vi "SPARC4_GEI.vi"() -> ()   [LabVIEW 2018]
uses:
  S4GEI/SPARC4_GEI.lvclass
  S4GEI/SPARC4_GEI.lvclass/SPARC4_GEI.ctl
  FWCS_ACS_Iterator/FWCS_ACS_Iterator.lvclass/FWCS_ACS_Iterator.ctl
  Interface/Interface.lvclass/Interface.ctl
  Channel GUI/Channel.lvclass/Channel.ctl
  State Machine/State Machine.lvclass/State Machine.ctl
  Filter_Wheel/Filter_Wheel.lvclass/Filter_Wheel.ctl
  Channel GUI/Channel.lvclass
  FWCS_ACS_Iterator/FWCS_ACS_Iterator.lvclass
  State Machine/State Machine.lvclass
  Filter_Wheel/Filter_Wheel.lvclass
  RxTx/RxTx.lvclass
  Interface/Interface.lvclass
panel:
  in  "Tab Control 2":T1(tab)
  out "Frames done":u16(slide)=1 max=2 scale=0.0..1.0
  in  "Channel ID":u16=1 min=1
  in  "FOCUS":bool caption="TEST"
  in  "TEST":bool
  in  "ZERO":bool caption="BIAS"
  in  "FLAT":bool
  in  "OBJECT":bool caption="SCIENCE"
  in  "DARK":bool caption="TEST"
  in  "Suffix:":string
  in  "Comment:":string="Go SPARC4!"
  in  "Filter":u16(ring)=1 items=["U"=1, "B"=2, "V"=3, "R"=4, "I"=5, "Clear"=6]
  out "Cubes done":u16(slide)=1 max=2 scale=0.0..1.0
  out "Exposing":bool
  in  "Dummy":bool
  out "Camera On/Off":bool
  in  "Abort Acquisition":bool
  in  "Stop Acquisition":bool
  in  "#Cubes":u32=1 min=1
  in  "#Frames":u16=1 min=1 max=1000
  in  "Send Message":bool
  out "Response:":string
  in  "Command:":string
  out "Last image":string
  out "CCD Status":string
  out "Frame exp time (s)":dbl
  out "Temperature":i16
  out "Serial Number":u16
  in  "Exposure Time (s)":dbl=1.0 min=9.999999747378752e-06
  in  "Acquire":bool
  in  "Stop Application":bool
  out "Error Message":string
  in  "Set camera configuration":bool
  in  "Cooler ON/OFF":u16(ring) items=["Cooler OFF", "Cooler ON"]
  in  "Temperature (ºC)":i16=20 min=-80 max=20
  in  "Set temperature":bool
  in  "Communication variables":T2={"FWCS IP"="200.131.64.49", "ACS IP"="200.131.64.49", "TCS COM Port"="COM1", "TCS Simulated/Real"=FALSE}
  in  "EM Gain":u16=2
  in  "EM Mode":u8(ring)=1 items=["Electron Multiplying", "Conventional"]
  in  "Readout Rate":u8(ring) items=["1 MHz", "0.1 MHz"]
  in  "Pre-amp gain":u8(ring) items=["Gain 1", "Gain 2"]
  in  "Vertical Clock Voltagem":u16(ring) items=["Normal", "+1", "+2", "+3", "+4"]
  in  "Acquisition Mode":u16(ring)=3 items=["Reserved", "Single Scan", "Accumulate", "Kinetic", "Fast Kinetic", "Run till abort", "Reserved", "Reserved", "Reserved", "Time Delayed Integration"]
  in  "Read Mode":u16(ring)=4 items=["Full Vertical Binning", "Multi-Track", "Random-Track", "Single-Track", "Image"]
  in  "Trigger Mode":u16(ring) items=["Internal", "External", "N/A", "N/A", "N/A", "N/A", "External Start", "External Exposure (Bulb)", "N/A", "External FVB EM", "Software", "N/A", "External Charge Shifting"]
  in  "Vertical Shift Speed":u16(ring)=3 items=["0.6", "1.13", "2.2", "4.33"]
  in  "AD Channel":u16
  in  "Shutter Mode":u8(ring)=2 items=["Fully Auto", "OPEN", "CLOSED"]
  in  "Shutter Time":u16=50
  in  "Shutter TTL":u16(ring) items=["TTL Low", "TTL High"]
  in  "Binning":u16=1
  in  "Initial Line":u16=1
  in  "Initial Cloumn":u16=1
  in  "Final Column":u16=1024
  in  "Final Line":u16=1024
  in  "Sub Image":T3(radio)=enum."1024 x 1024"
  in  "Frame Tansfer":bool=TRUE
  in  "stop iterations":bool
  out "Exposing 2":bool
  out "Frame exp time (s) \n2":dbl
  out "Exposições realizadas 2":u16(slide)=1 max=2
  in  "Acquisition configuration 6":T4={"Select"=FALSE, "Exp Time"=1.0, "#Frames"=1, "Sufix"="", "Filter"=6} {"Filter" items=["U"=1, "B"=2, "V"=3, "R"=4, "I"=5, "Clear"=6]}
  in  "Acquisition configuration 5":T4={"Select"=FALSE, "Exp Time"=1.0, "#Frames"=1, "Sufix"="", "Filter"=5} {"Filter" items=["U"=1, "B"=2, "V"=3, "R"=4, "I"=5, "Clear"=6]}
  in  "Acquisition configuration 4":T4={"Select"=FALSE, "Exp Time"=1.0, "#Frames"=1, "Sufix"="", "Filter"=4} {"Filter" items=["U"=1, "B"=2, "V"=3, "R"=4, "I"=5, "Clear"=6]}
  in  "Acquisition configuration 3":T4={"Select"=FALSE, "Exp Time"=1.0, "#Frames"=1, "Sufix"="", "Filter"=3} {"Filter" items=["U"=1, "B"=2, "V"=3, "R"=4, "I"=5, "Clear"=6]}
  in  "Acquisition configuration 2":T4={"Select"=FALSE, "Exp Time"=1.0, "#Frames"=1, "Sufix"="", "Filter"=2} {"Filter" items=["U"=1, "B"=2, "V"=3, "R"=4, "I"=5, "Clear"=6]}
  in  "Number of iterations":u16=1
  out "Current filter":u16(ring)=1 items=["U"=1, "B"=2, "V"=3, "R"=4, "I"=5, "Clear"=6]
  in  "Start Iterations":bool
  out "Iterations Done":u16(slide) scale=0.0..1.0
  in  "Acquisition configuration":T4={"Select"=FALSE, "Exp Time"=1.0, "#Frames"=1, "Sufix"="", "Filter"=1} {"Filter" items=["U"=1, "B"=2, "V"=3, "R"=4, "I"=5, "Clear"=6]}
  # "SPARC4  ACS\nGraphical Engineering Interface (GEI)"
  # "FWCS Iterator"
  # "Select"
  # "Filter"
  # "#Frames"
  # "Exp time (s)"
  # "Suffix"
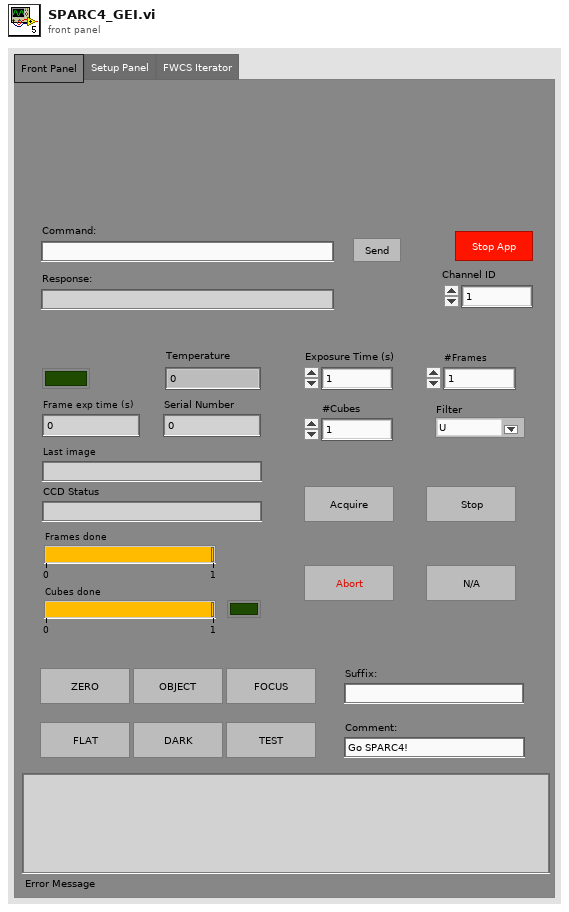
[diagram p1: front panel]
types:
  T1 = enum32{"Front Panel", "Setup Panel", "FWCS Iterator"}
  T2 = cluster{"FWCS IP":string, "ACS IP":string, "TCS COM Port":string, "TCS Simulated/Real":bool}
  T3 = enum32{"256 x 256", "512 x 512", "1024 x 1024", "Custom"}
  T4 = cluster{"Select":bool, "Exp Time":dbl, "#Frames":u16, "Sufix":string, "Filter":u16}
  T5 = enum8{"Enabled", "Disabled", "Disabled and Grayed Out"}
  T6 = cluster{"CUBE_EXPOSURE_TIME":sgl, "CUBES_DONE":u16, "LAST_IMAGE_NAME":string, "DISK_SPACE":u16, "FRAMES_DONE":u16, "CCD_STATUS":string, "CURRENT_TEMPERATURE":i16, "TEMPERATURE_STATUS":string, "FRAME_EXPOSURE_TIME":sgl, "CCD_POWER_STATUS":bool, "SERIAL_NUMBER":u16, "ACQUIRING":bool}
  T7 = cluster{"PREAMP":u16, "READOUT_RATE":u16, "EM_GAIN":u16, "VBIN":u16, "INITIAL_LINE":u16, "INITIAL_COLUMN":u16, "FINAL_LINE":u16, "FINAL_COLUMN":u16, "TRIGGER_MODE":u16, "HBIN":u16, "SHUTTER_TTL":u16, "SHUTTER_MODE":u16, "SHUTTER_OPENING_TIME":u16, "SHUTTER_CLOSING_TIME":u16, "VERTICAL_SHIFT_SPEED":u16, "READ_MODE":u16, "FRAME_TRANSFER":bool, "VERTICAL_CLOCK_VOLTAGE":u16, "ACQUISITION_MODE":u16, "AD_CHANNEL":u16, "EM_MODE":u16}
  T8 = cluster{"COOLER_POWER_STATUS":u16, "TEMP":i32, "EXPTIME":sgl, "#FRAMES":u32, "#CUBES":u32}
  T9 = cluster{"Select":bool, "Exp Time":dbl, "#Frames":u16, "Sufix":string, "Filter":u16}[]
  T10 = cluster{"Select":bool, "Exp Time":u16, "#Frames":u16, "Sufix":string, "Filter":u16}
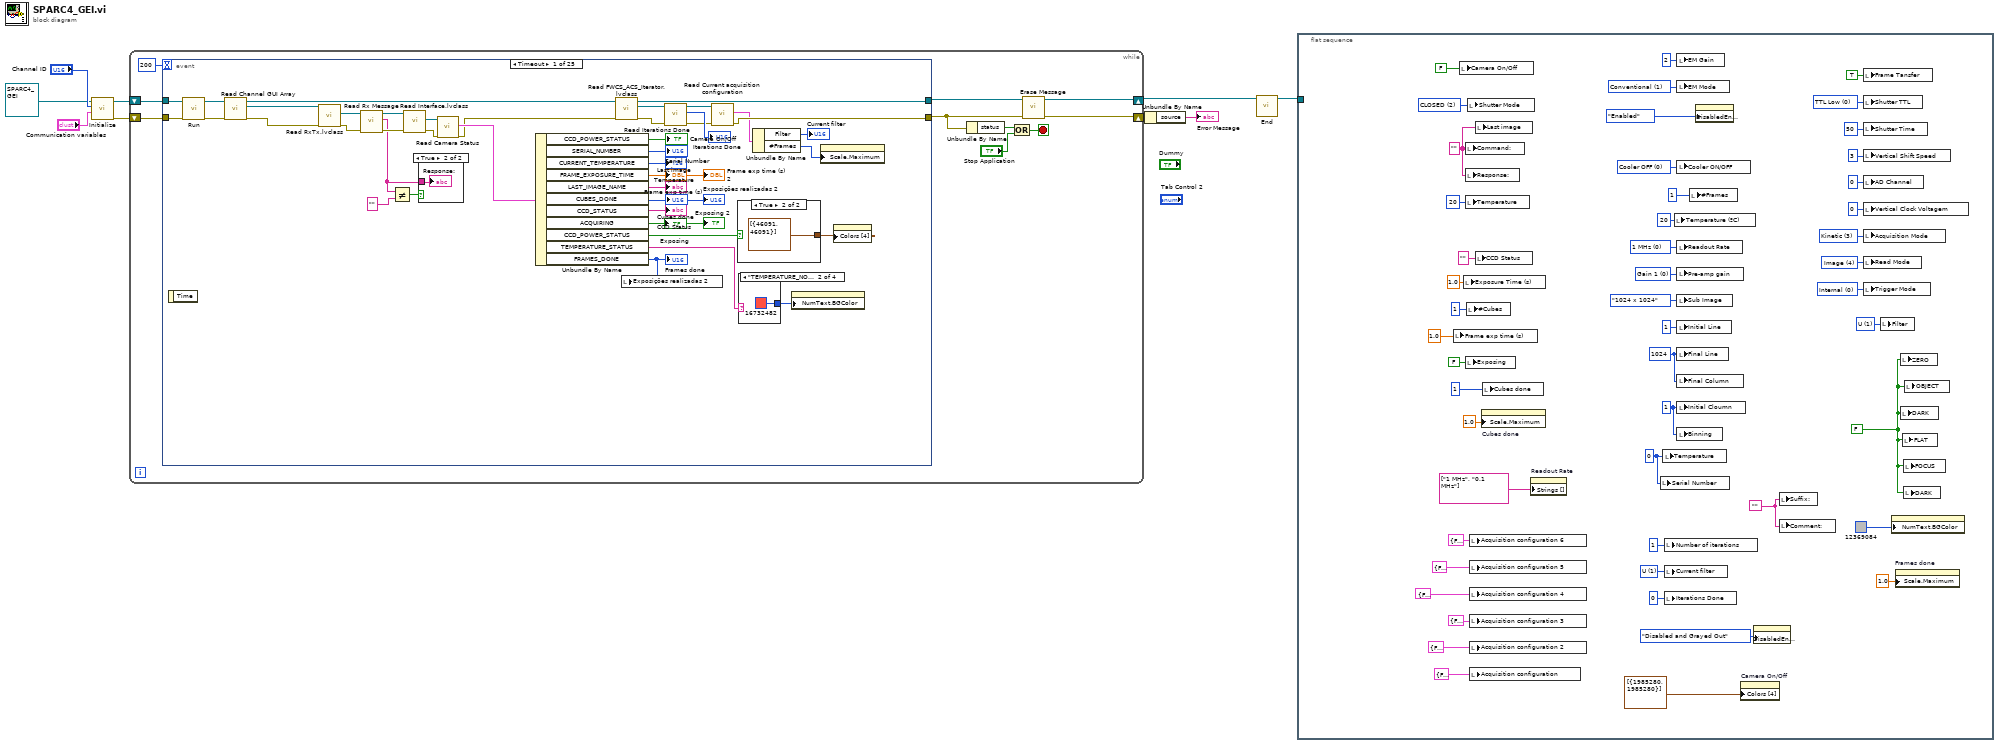
[diagram p0: block diagram]
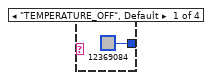
[diagram p2: hidden frame]
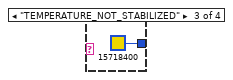
[diagram p3: hidden frame]
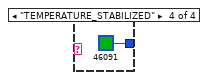
[diagram p4: hidden frame]
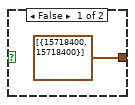
[diagram p5: hidden frame]
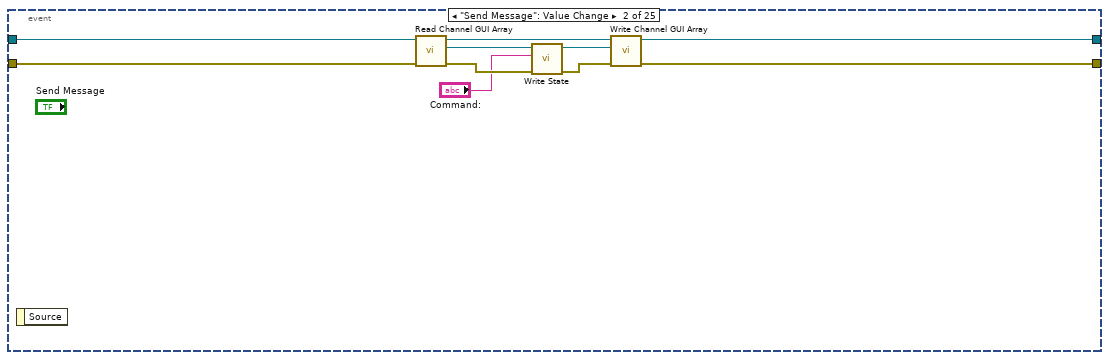
[diagram p7: hidden frame]
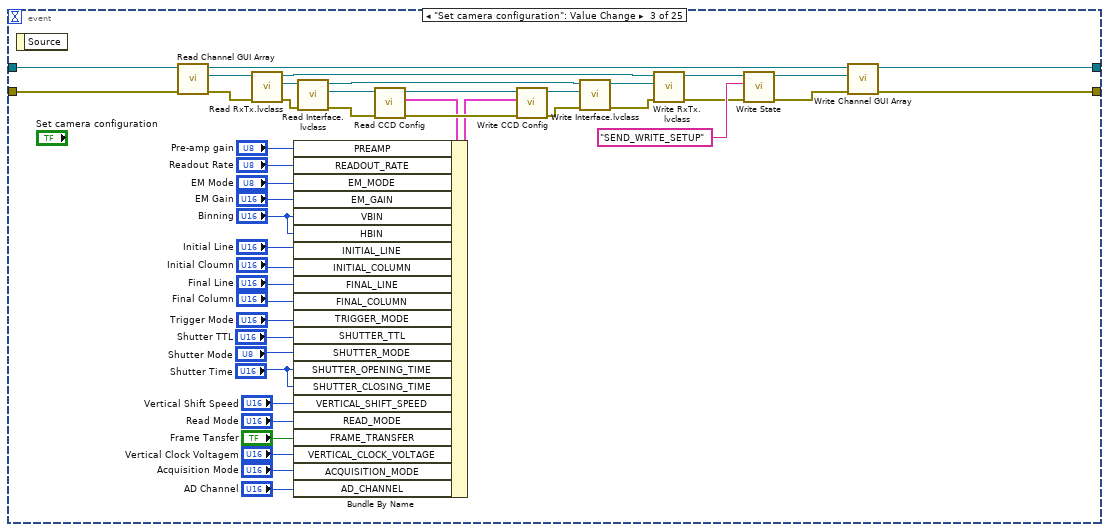
[diagram p8: hidden frame]
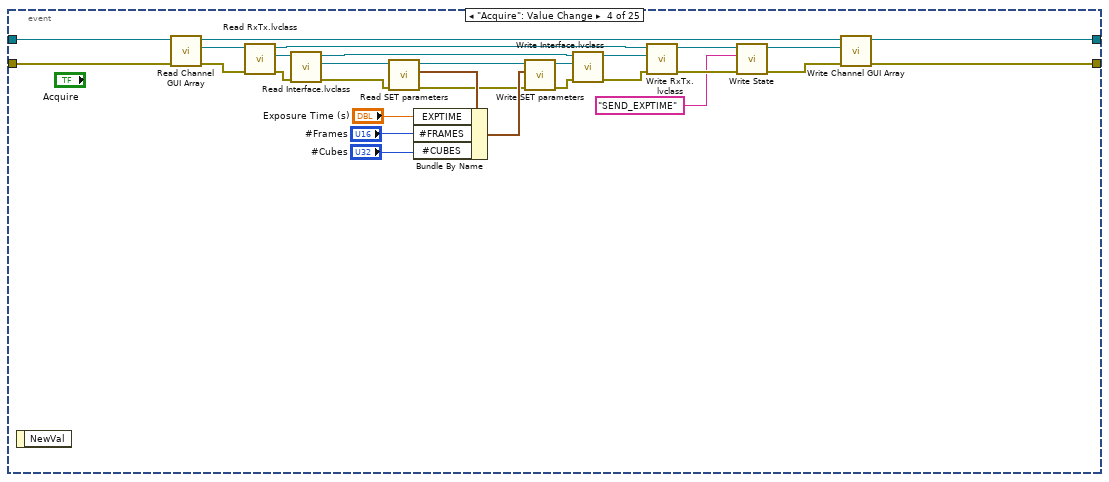
[diagram p9: hidden frame]
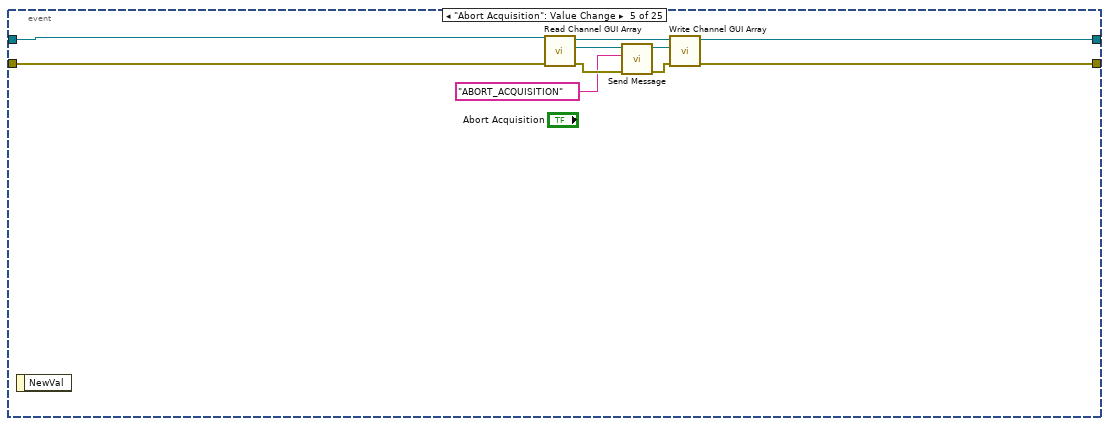
[diagram p10: hidden frame]
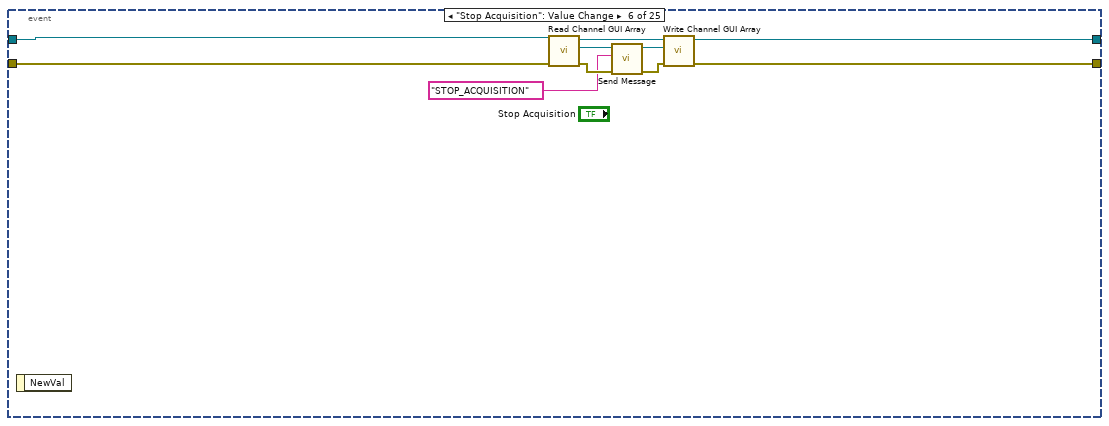
[diagram p11: hidden frame]
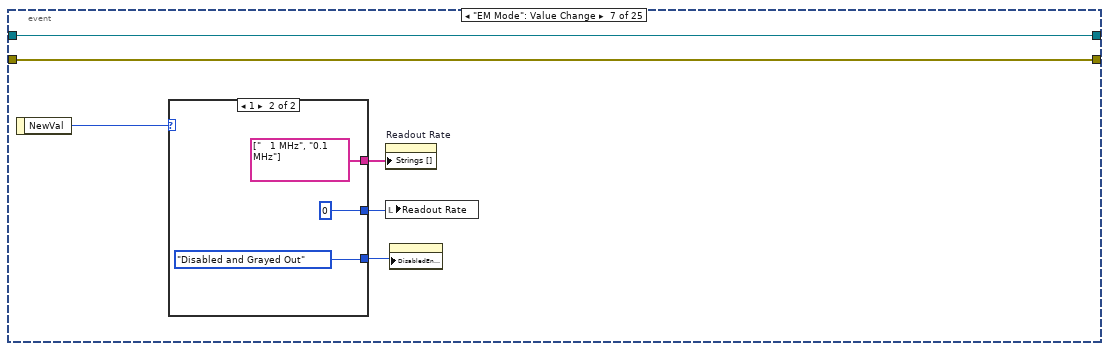
[diagram p12: hidden frame]
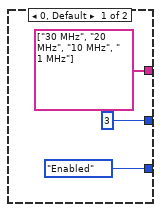
[diagram p13: hidden frame]
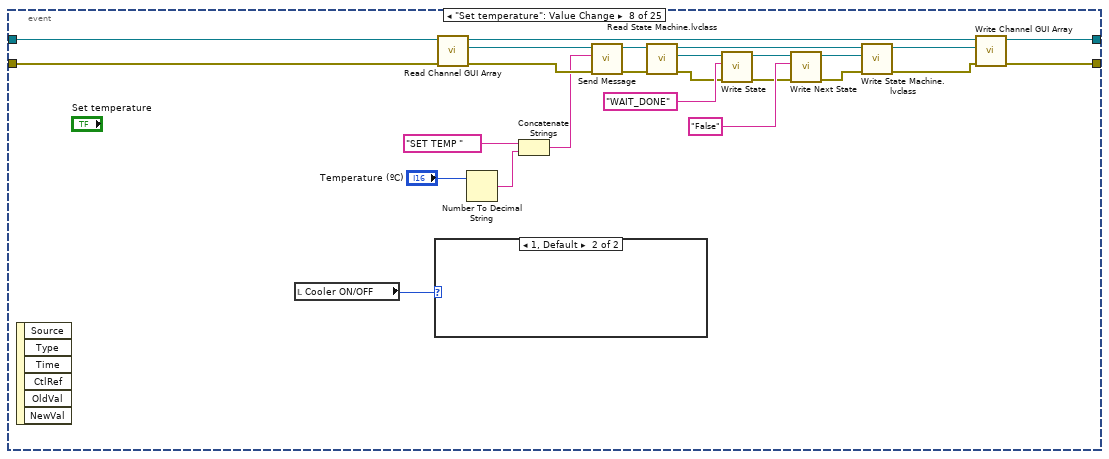
[diagram p14: hidden frame]
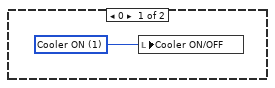
[diagram p15: hidden frame]
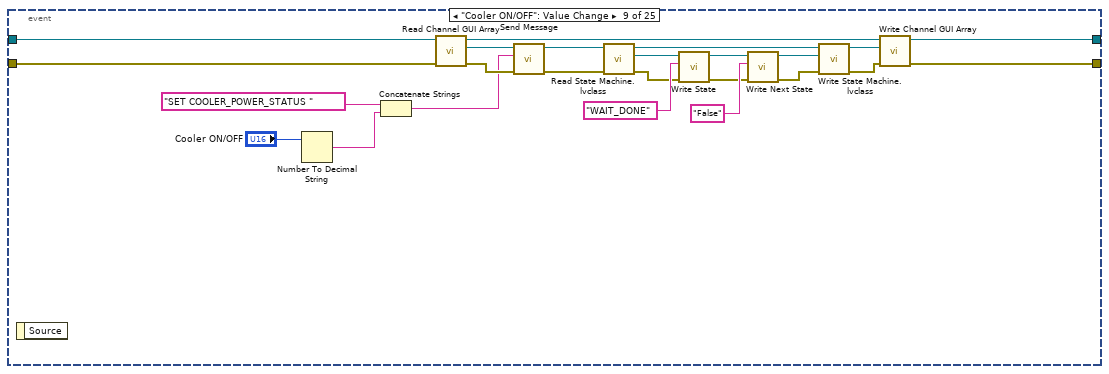
[diagram p16: hidden frame]
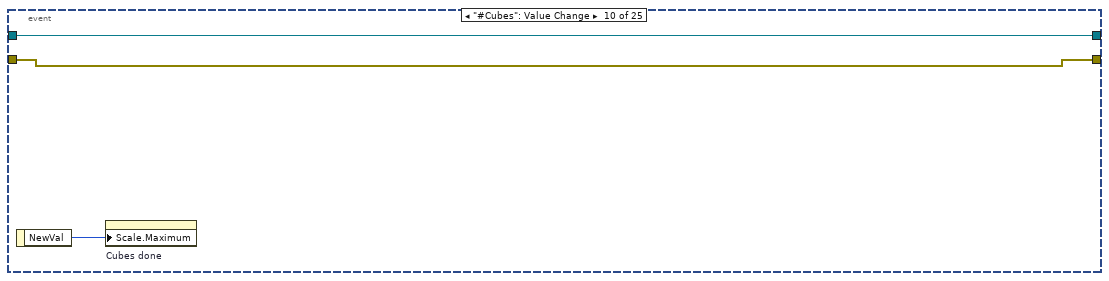
[diagram p17: hidden frame]
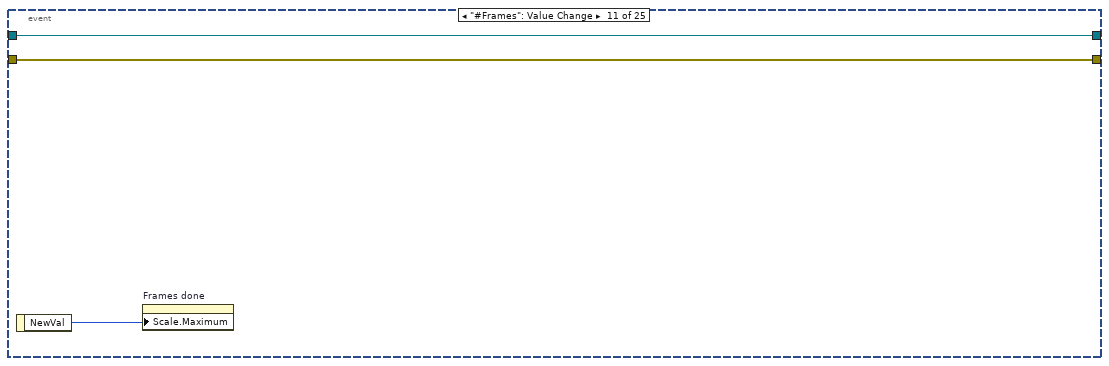
[diagram p18: hidden frame]
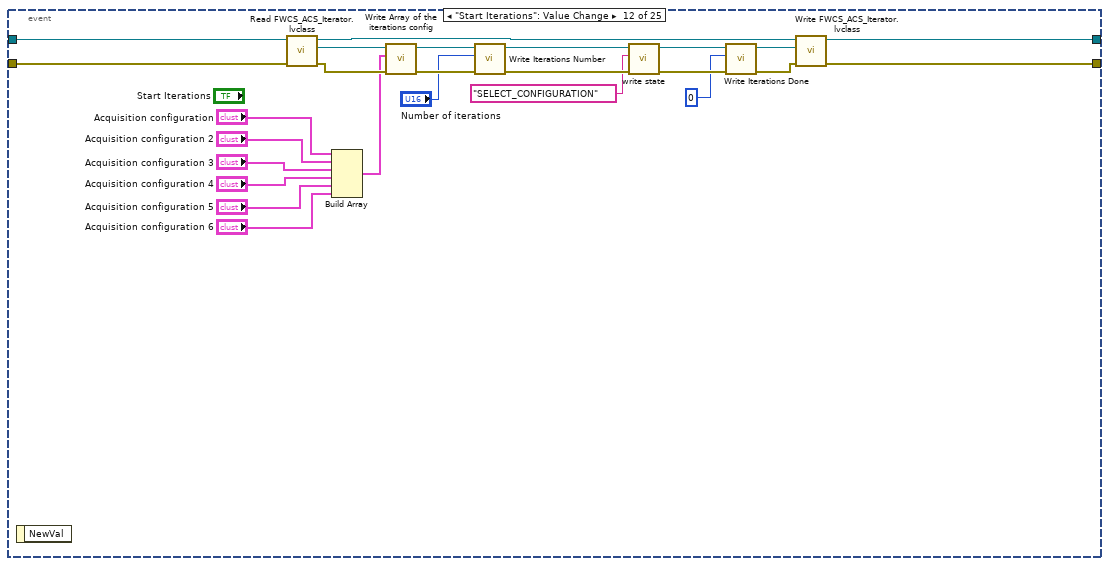
[diagram p19: hidden frame]
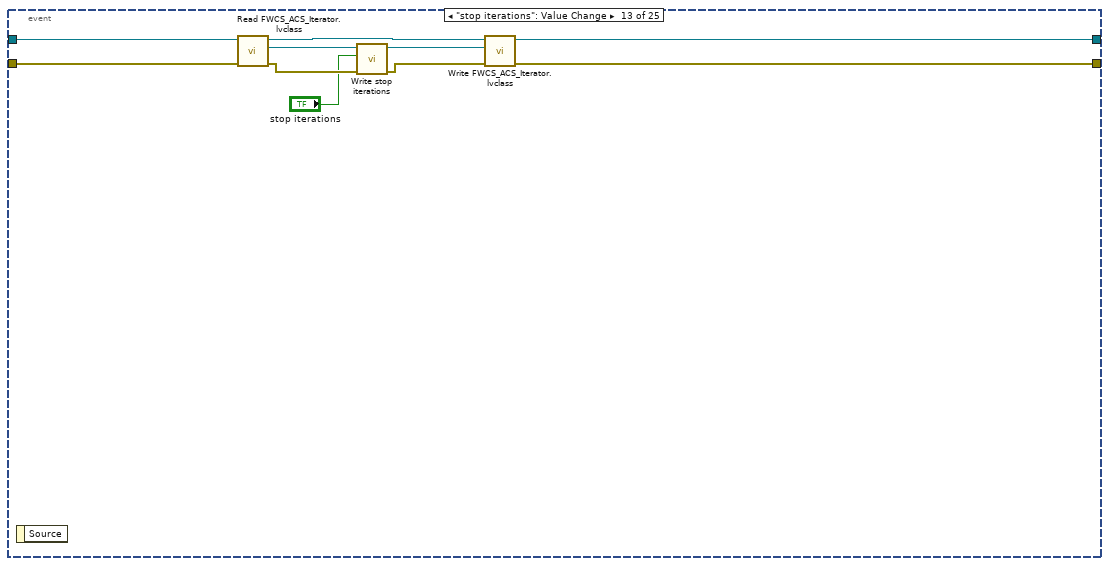
[diagram p20: hidden frame]
diagram:
  n1 = call "Initialize.vi"("Communication variables"="Communication variables", "Channel ID"="Channel ID", "SPARC4_GUI in"=refnum<class "SPARC4_GEI.lvclass"> refnum ("SPARC4_GUI.lvclass")) -> ("error out"=w9:errorcluster, "SPARC4_GUI out"=w8:refnum<class "SPARC4_GEI.lvclass">)  [unwired: 7 in]
  n2 = while {
    shift-right: [w13] -> w5
    shift-left: w9 -> [w14]
    shift-right: [w12] -> w6
    shift-left: w8 -> [w15]
    stop <- w18 stop-if-true
    n3 = event shown="[0] Timeout" {
      selector: _ -> [_ _ _ _ _ _ _ _ _ _ _ _ _ _ _ _ _ _ _ _ _ _ _ _ _]
      dyn-events: _ -> [_ _ _ _ _ _ _ _ _ _ _ _ _ _ _ _ _ _ _ _ _ _ _ _ _]
      timeout: 200 -> [_ _ _ _ _ _ _ _ _ _ _ _ _ _ _ _ _ _ _ _ _ _ _ _ _]
      tunnel: w14 -> [w57 w76 w121 w127 w156 w166 w176 w199 w225 w235 w237 w263 w273 w276 w294 w329 w352 w387 w417 w449 w480 w511 w540 w556 w560]
      tunnel: [w32 w69 w115 w125 w154 w164 w176 w204 w223 w235 w237 w261 w271 w276 w292 w327 w350 w385 w415 w447 w478 w509 w538 w544 w560] -> w10
      tunnel: w15 -> [w58 w77 w122 w128 w157 w167 w177 w198 w226 w236 w238 w264 w274 w277 w295 w330 w353 w388 w418 w450 w481 w512 w541 w555 w559]
      tunnel: [w36 w70 w116 w126 w155 w165 w177 w205 w224 w236 w238 w262 w272 w277 w293 w328 w351 w386 w416 w448 w479 w510 w539 w545 w559] -> w11
      event Timeout {
        n4 = event-data() -> ()  [unwired: 1 in, 1 out]
        n5 = call "Run.vi"("error in (no error)"=w57, "SPARC4_GUI in"=w58) -> ("error out"=w60:errorcluster, "SPARC4_GUI out"=w59:refnum<class "SPARC4_GEI.lvclass">)  [unwired: 8 in]
        n6 = call "Read Channel GUI Array.vi"("error in (no error)"=w60, "SPARC4_GUI in"=w59) -> ("error out"=w54:errorcluster, "Channel.lvclass"=w25:refnum<class "Channel.lvclass">, "SPARC4_GUI out"=w40:refnum<class "SPARC4_GEI.lvclass">)  [unwired: 7 in]
        n7 = call "Read RxTx.lvclass.vi"("error in (no error)"=w54, "Channel GUI in"=w25) -> ("error out"=w53:errorcluster, "RxTx.lvclass"=w52:refnum<class "RxTx.lvclass">)  [unwired: 7 in, 1 out]
        n8 = call "Read Rx Message.vi"("error in (no error)"=w53, "RxTx in"=w52) -> ("error out"=w55:errorcluster, "Rx Message"=w42:string, "RxTx out"=w56:refnum<class "RxTx.lvclass">)  [unwired: 7 in]
        n9 = Not Equal?(x=w42, y="") -> (x != y?=w43:bool)
        n10 = call "Read Interface.lvclass.vi"("error in (no error)"=w55, "RxTx in"=w56) -> ("error out"=w45:errorcluster, "Interface.lvclass"=w46:refnum<class "Interface.lvclass">)  [unwired: 7 in, 1 out]
        n11 = case shown="True" w43 {
          tunnel: w42 -> [_ w67]
          frame False {
          }
          frame True {
            "Response:" <- w67
          }
        }
        n12 = call "Read Camera Status.vi"("error in (no error)"=w45, "Interface in"=w46) -> ("error out"=w39:errorcluster, "Camera Status"=w44:T6)  [unwired: 7 in, 1 out]
        n13 = Unbundle By Name(w44) -> ("CCD_POWER_STATUS"=→"Camera On/Off":bool, "SERIAL_NUMBER"=→"Serial Number":u16, "CURRENT_TEMPERATURE"=→"Temperature":i16, "FRAME_EXPOSURE_TIME"=→"Frame exp time (s)" →"Frame exp time (s) \n2":sgl, "LAST_IMAGE_NAME"=→"Last image":string, "CUBES_DONE"=→"Cubes done" →"Exposições realizadas 2":u16, "CCD_STATUS"=→"CCD Status":string, "ACQUIRING"=→"Exposing" →"Exposing 2":bool, "CCD_POWER_STATUS"=w23:bool, "TEMPERATURE_STATUS"=w22:string, "FRAMES_DONE"=w20:u16)
        "Frames done" <- w20
        n14 = call "Read FWCS_ACS_Iterator.lvclass.vi"("error in (no error)"=w39, "SPARC4_GEI in"=w40) -> ("error out"=w37:errorcluster, "FWCS_ACS_Iterator.lvclass"=w38:refnum<class "FWCS_ACS_Iterator.lvclass">, "SPARC4_GEI out"=w36:refnum<class "SPARC4_GEI.lvclass">)  [unwired: 7 in]
        n15 = local write "Exposições realizadas 2"(w20) -> ()
        n16 = call "Read Iterations Done.vi"("error in (no error)"=w37, "FWCS_ACS_Iterator in"=w38) -> ("error out"=w34:errorcluster, "Iterations Done"=→"Iterations Done":u16, "FWCS_ACS_Iterator out"=w33:refnum<class "FWCS_ACS_Iterator.lvclass">)  [unwired: 7 in]
        n17 = call "Read Current acquisition configuration.vi"("error in (no error)"=w34, "FWCS_ACS_Iterator in"=w33) -> ("error out"=w32:errorcluster, "Current acquisition configuration"=w31:T4)  [unwired: 7 in, 1 out]
        n18 = case shown="True" w23 {
          tunnel: [cluster{u32, u32}[] [{15718400, 15718400}] ("Colors [4]") cluster{u32, u32}[] [{46091, 46091}] ("Colors [4]")] -> w24
          frame False {
          }
          frame True {
          }
        }
        n19 = case shown="\"TEMPERATURE_NOT_REACHED\"" w22 {
          tunnel: [u32 12369084 u32 16732482 u32 15718400 u32 46091] -> w21
          frame "TEMPERATURE_OFF", Default {
          }
          frame "TEMPERATURE_NOT_REACHED" {
          }
          frame "TEMPERATURE_NOT_STABILIZED" {
          }
          frame "TEMPERATURE_STABILIZED" {
          }
        }
        n20 = Unbundle By Name(w31) -> ("Filter"=→"Current filter":u16, "#Frames"=w26:u16)
        n21 = property on="Temperature" class="DigNum (strict)"("NumText.BGColor"=w21) -> ()  [unwired: 2 in, 2 out]
        n22 = property on="Exposições realizadas 2" class="Slide (strict)"("Scale.Maximum"=w26) -> ()  [unwired: 2 in, 2 out]
        n23 = property on="Camera On/Off" class="Bool (strict)"("Colors [4]"=w24) -> ()  [unwired: 2 in, 2 out]
      }
      event "Send Message": Value Change {
        n24 = event-data() -> ()  [unwired: 1 in, 1 out]
        n25 = call "Read Channel GUI Array.vi"("error in (no error)"=w76, "SPARC4_GUI in"=w77) -> ("error out"=w73:errorcluster, "Channel.lvclass"=w75:refnum<class "Channel.lvclass">, "SPARC4_GUI out"=w72:refnum<class "SPARC4_GEI.lvclass">)  [unwired: 7 in]
        n26 = call "Write State.vi"("error in (no error)"=w73, "State"="Command:", "Channel GEI in"=w75) -> ("error out"=w74:errorcluster, "Channel GEI out"=w68:refnum<class "Channel.lvclass">)  [unwired: 7 in]
        n27 = call "Write Channel GUI Array.vi"("error in (no error)"=w74, "Channel.lvclass"=w68, "SPARC4_GUI in"=w72) -> ("error out"=w69:errorcluster, "SPARC4_GUI out"=w70:refnum<class "SPARC4_GEI.lvclass">)  [unwired: 7 in]
      }
      event "Set camera configuration": Value Change {
        n28 = event-data() -> ()  [unwired: 1 in, 1 out]
        n29 = call "Read Channel GUI Array.vi"("error in (no error)"=w121, "SPARC4_GUI in"=w122) -> ("error out"=w119:errorcluster, "Channel.lvclass"=w120:refnum<class "Channel.lvclass">, "SPARC4_GUI out"=w117:refnum<class "SPARC4_GEI.lvclass">)  [unwired: 7 in]
        n30 = call "Read RxTx.lvclass.vi"("error in (no error)"=w119, "Channel GUI in"=w120) -> ("error out"=w114:errorcluster, "RxTx.lvclass"=w113:refnum<class "RxTx.lvclass">, "Channel GUI out"=w78:refnum<class "Channel.lvclass">)  [unwired: 7 in]
        n31 = call "Read Interface.lvclass.vi"("error in (no error)"=w114, "RxTx in"=w113) -> ("error out"=w108:errorcluster, "Interface.lvclass"=w111:refnum<class "Interface.lvclass">, "RxTx out"=w83:refnum<class "RxTx.lvclass">)  [unwired: 7 in]
        n32 = call "Read CCD Config.vi"("error in (no error)"=w108, "Interface in"=w111) -> ("error out"=w109:errorcluster, "CCD Config"=w89:T7, "Interface out"=w110:refnum<class "Interface.lvclass">)  [unwired: 7 in]
        n33 = Bundle By Name(cluster=w89, "PREAMP"="Pre-amp gain", "READOUT_RATE"="Readout Rate", "EM_MODE"="EM Mode", "EM_GAIN"="EM Gain", "VBIN"="Binning", "HBIN"="Binning", "INITIAL_LINE"="Initial Line", "INITIAL_COLUMN"="Initial Cloumn", "FINAL_LINE"="Final Line", "FINAL_COLUMN"="Final Column", "TRIGGER_MODE"="Trigger Mode", "SHUTTER_TTL"="Shutter TTL", "SHUTTER_MODE"="Shutter Mode", "SHUTTER_OPENING_TIME"="Shutter Time", "SHUTTER_CLOSING_TIME"="Shutter Time", "VERTICAL_SHIFT_SPEED"="Vertical Shift Speed", "READ_MODE"="Read Mode", "FRAME_TRANSFER"="Frame Tansfer", "VERTICAL_CLOCK_VOLTAGE"="Vertical Clock Voltagem", "ACQUISITION_MODE"="Acquisition Mode", "AD_CHANNEL"="AD Channel") -> (w88:T7)
        n34 = call "Write CCD Config.vi"("error in (no error)"=w109, "CCD Config"=w88, "Interface in"=w110) -> ("error out"=w84:errorcluster, "Interface out"=w85:refnum<class "Interface.lvclass">)  [unwired: 7 in]
        n35 = call "Write Interface.lvclass.vi"("error in (no error)"=w84, "Interface.lvclass"=w85, "RxTx in"=w83) -> ("error out"=w81:errorcluster, "RxTx out"=w82:refnum<class "RxTx.lvclass">)  [unwired: 7 in]
        n36 = call "Write RxTx.lvclass.vi"("error in (no error)"=w81, "RxTx.lvclass"=w82, "Channel GUI in"=w78) -> ("error out"=w80:errorcluster, "Channel GUI out"=w79:refnum<class "Channel.lvclass">)  [unwired: 7 in]
        n37 = call "Write State.vi"("error in (no error)"=w80, "State"="SEND_WRITE_SETUP", "Channel GEI in"=w79) -> ("error out"=w118:errorcluster, "Channel GEI out"=w86:refnum<class "Channel.lvclass">)  [unwired: 7 in]
        n38 = call "Write Channel GUI Array.vi"("error in (no error)"=w118, "Channel.lvclass"=w86, "SPARC4_GUI in"=w117) -> ("error out"=w115:errorcluster, "SPARC4_GUI out"=w116:refnum<class "SPARC4_GEI.lvclass">)  [unwired: 7 in]
      }
      event "Acquire": Value Change {
        n39 = event-data() -> ()  [unwired: 1 in, 1 out]
        n40 = call "Read Channel GUI Array.vi"("error in (no error)"=w127, "SPARC4_GUI in"=w128) -> ("error out"=w142:errorcluster, "Channel.lvclass"=w143:refnum<class "Channel.lvclass">, "SPARC4_GUI out"=w140:refnum<class "SPARC4_GEI.lvclass">)  [unwired: 7 in]
        n41 = call "Read RxTx.lvclass.vi"("error in (no error)"=w142, "Channel GUI in"=w143) -> ("error out"=w139:errorcluster, "RxTx.lvclass"=w138:refnum<class "RxTx.lvclass">, "Channel GUI out"=w131:refnum<class "Channel.lvclass">)  [unwired: 7 in]
        n42 = call "Read Interface.lvclass.vi"("error in (no error)"=w139, "RxTx in"=w138) -> ("error out"=w145:errorcluster, "Interface.lvclass"=w144:refnum<class "Interface.lvclass">, "RxTx out"=w136:refnum<class "RxTx.lvclass">)  [unwired: 7 in]
        n43 = call "Read SET parameters.vi"("error in (no error)"=w145, "Interface in"=w144) -> ("error out"=w148:errorcluster, "SET parameters"=w150:T8, "Interface out"=w149:refnum<class "Interface.lvclass">)  [unwired: 7 in]
        n44 = Bundle By Name(cluster=w150, "EXPTIME"="Exposure Time (s)", "#FRAMES"="#Frames", "#CUBES"="#Cubes") -> (w151:T8)
        n45 = call "Write SET parameters.vi"("error in (no error)"=w148, "SET parameters"=w151, "Interface in"=w149) -> ("error out"=w147:errorcluster, "Interface out"=w146:refnum<class "Interface.lvclass">)  [unwired: 7 in]
        n46 = call "Write Interface.lvclass.vi"("error in (no error)"=w147, "Interface.lvclass"=w146, "RxTx in"=w136) -> ("error out"=w134:errorcluster, "RxTx out"=w135:refnum<class "RxTx.lvclass">)  [unwired: 7 in]
        n47 = call "Write RxTx.lvclass.vi"("error in (no error)"=w134, "RxTx.lvclass"=w135, "Channel GUI in"=w131) -> ("error out"=w133:errorcluster, "Channel GUI out"=w132:refnum<class "Channel.lvclass">)  [unwired: 7 in]
        n48 = call "Write State.vi"("error in (no error)"=w133, "State"="SEND_EXPTIME", "Channel GEI in"=w132) -> ("error out"=w141:errorcluster, "Channel GEI out"=w137:refnum<class "Channel.lvclass">)  [unwired: 7 in]
        n49 = call "Write Channel GUI Array.vi"("error in (no error)"=w141, "Channel.lvclass"=w137, "SPARC4_GUI in"=w140) -> ("error out"=w125:errorcluster, "SPARC4_GUI out"=w126:refnum<class "SPARC4_GEI.lvclass">)  [unwired: 7 in]
      }
      event "Abort Acquisition": Value Change {
        n50 = event-data() -> ()  [unwired: 1 in, 1 out]
        n51 = call "Read Channel GUI Array.vi"("error in (no error)"=w156, "SPARC4_GUI in"=w157) -> ("error out"=w158:errorcluster, "Channel.lvclass"=w160:refnum<class "Channel.lvclass">, "SPARC4_GUI out"=w161:refnum<class "SPARC4_GEI.lvclass">)  [unwired: 7 in]
        n52 = call "Send Message.vi"("error in (no error)"=w158, "Message"="ABORT_ACQUISITION", "Channel GUI in"=w160) -> ("error out"=w159:errorcluster, "Channel GUI out"=w152:refnum<class "Channel.lvclass">)  [unwired: 7 in]
        n53 = call "Write Channel GUI Array.vi"("error in (no error)"=w159, "Channel.lvclass"=w152, "SPARC4_GUI in"=w161) -> ("error out"=w154:errorcluster, "SPARC4_GUI out"=w155:refnum<class "SPARC4_GEI.lvclass">)  [unwired: 7 in]
      }
      event "Stop Acquisition": Value Change {
        n54 = event-data() -> ()  [unwired: 1 in, 1 out]
        n55 = call "Read Channel GUI Array.vi"("error in (no error)"=w166, "SPARC4_GUI in"=w167) -> ("error out"=w168:errorcluster, "Channel.lvclass"=w170:refnum<class "Channel.lvclass">, "SPARC4_GUI out"=w171:refnum<class "SPARC4_GEI.lvclass">)  [unwired: 7 in]
        n56 = call "Send Message.vi"("error in (no error)"=w168, "Message"="STOP_ACQUISITION", "Channel GUI in"=w170) -> ("error out"=w169:errorcluster, "Channel GUI out"=w162:refnum<class "Channel.lvclass">)  [unwired: 7 in]
        n57 = call "Write Channel GUI Array.vi"("error in (no error)"=w169, "Channel.lvclass"=w162, "SPARC4_GUI in"=w171) -> ("error out"=w164:errorcluster, "SPARC4_GUI out"=w165:refnum<class "SPARC4_GEI.lvclass">)  [unwired: 7 in]
      }
      event "EM Mode": Value Change {
        n58 = event-data() -> ("NewVal"=w174:u8)  [unwired: 1 in]
        n59 = case shown="1" w174 {
          tunnel: [string[] ["30 MHz", "20 MHz", "10 MHz", "  1 MHz"] string[] ["   1 MHz", "0.1 MHz"]] -> w175
          tunnel: [3 0] -> w173
          tunnel: [T5."Enabled" ("Disabled") T5."Disabled and Grayed Out" ("Disabled")] -> w172
          frame 0, Default {
          }
          frame 1 {
          }
        }
        n60 = property on="Readout Rate" class="Ring (strict)"("Strings []"=w175) -> ()  [unwired: 2 in, 2 out]
        n61 = local write "Readout Rate"(w173) -> ()
        n62 = property on="EM Gain" class="DigNum (strict)"("DisabledEnum"=w172) -> ()  [unwired: 2 in, 2 out]
      }
      event "Set temperature": Value Change {
        n63 = event-data() -> ()  [unwired: 1 in, 6 out]
        n64 = local read "Cooler ON/OFF"() -> (w184:u16)
        n65 = case shown="1, Default" w184 {
          frame 0 {
            w209 = u16 1 items=["Cooler OFF", "Cooler ON"] ("Cooler ON/OFF")
            n66 = local write "Cooler ON/OFF"(w209) -> ()
          }
          frame 1, Default {
          }
        }
        n67 = call "Read Channel GUI Array.vi"("error in (no error)"=w199, "SPARC4_GUI in"=w198) -> ("error out"=w200:errorcluster, "Channel.lvclass"=w201:refnum<class "Channel.lvclass">, "SPARC4_GUI out"=w202:refnum<class "SPARC4_GEI.lvclass">)  [unwired: 7 in]
        n68 = Number To Decimal String(number="Temperature (ºC)") -> (decimal integer string=w207:string)  [unwired: 1 in]
        n69 = Concatenate Strings("SET TEMP " ("Message"), w207) -> (w197:string)
        n70 = call "Send Message.vi"("error in (no error)"=w200, "Message"=w197, "Channel GUI in"=w201) -> ("error out"=w193:errorcluster, "Channel GUI out"=w194:refnum<class "Channel.lvclass">)  [unwired: 7 in]
        n71 = call "Read State Machine.lvclass.vi"("error in (no error)"=w193, "Channel GUI in"=w194) -> ("error out"=w187:errorcluster, "State Machine.lvclass"=w192:refnum<class "State Machine.lvclass">, "Channel GUI out"=w186:refnum<class "Channel.lvclass">)  [unwired: 7 in]
        n72 = call-dynamic "Write State.vi"("error in (no error)"=w187, "State"="WAIT_DONE" ("Message"), "State Machine in"=w192) -> ("error out"=w188:errorcluster, "State Machine out"=w191:refnum<class "State Machine.lvclass">)  [unwired: 7 in]
        n73 = call "Write Next State.vi"("error in (no error)"=w188, "Next State"="False" ("Message"), "State Machine in"=w191) -> ("error out"=w189:errorcluster, "State Machine out"=w190:refnum<class "State Machine.lvclass">)  [unwired: 7 in]
        n74 = call "Write State Machine.lvclass.vi"("error in (no error)"=w189, "State Machine.lvclass"=w190, "Channel GUI in"=w186) -> ("error out"=w203:errorcluster, "Channel GUI out"=w185:refnum<class "Channel.lvclass">)  [unwired: 7 in]
        n75 = call "Write Channel GUI Array.vi"("error in (no error)"=w203, "Channel.lvclass"=w185, "SPARC4_GUI in"=w202) -> ("error out"=w204:errorcluster, "SPARC4_GUI out"=w205:refnum<class "SPARC4_GEI.lvclass">)  [unwired: 7 in]
      }
      event "Cooler ON/OFF": Value Change {
        n76 = event-data() -> ()  [unwired: 1 in, 1 out]
        n77 = Number To Decimal String(number="Cooler ON/OFF") -> (decimal integer string=w231:string)  [unwired: 1 in]
        n78 = Concatenate Strings("SET COOLER_POWER_STATUS ", w231) -> (w222:string)
        n79 = call "Read Channel GUI Array.vi"("error in (no error)"=w225, "SPARC4_GUI in"=w226) -> ("error out"=w227:errorcluster, "Channel.lvclass"=w228:refnum<class "Channel.lvclass">, "SPARC4_GUI out"=w229:refnum<class "SPARC4_GEI.lvclass">)  [unwired: 7 in]
        n80 = call "Send Message.vi"("error in (no error)"=w227, "Message"=w222, "Channel GUI in"=w228) -> ("error out"=w211:errorcluster, "Channel GUI out"=w212:refnum<class "Channel.lvclass">)  [unwired: 7 in]
        n81 = call "Read State Machine.lvclass.vi"("error in (no error)"=w211, "Channel GUI in"=w212) -> ("error out"=w218:errorcluster, "State Machine.lvclass"=w213:refnum<class "State Machine.lvclass">, "Channel GUI out"=w219:refnum<class "Channel.lvclass">)  [unwired: 7 in]
        n82 = call-dynamic "Write State.vi"("error in (no error)"=w218, "State"="WAIT_DONE" ("Message"), "State Machine in"=w213) -> ("error out"=w217:errorcluster, "State Machine out"=w214:refnum<class "State Machine.lvclass">)  [unwired: 7 in]
        n83 = call "Write Next State.vi"("error in (no error)"=w217, "Next State"="False" ("Message"), "State Machine in"=w214) -> ("error out"=w216:errorcluster, "State Machine out"=w215:refnum<class "State Machine.lvclass">)  [unwired: 7 in]
        n84 = call "Write State Machine.lvclass.vi"("error in (no error)"=w216, "State Machine.lvclass"=w215, "Channel GUI in"=w219) -> ("error out"=w230:errorcluster, "Channel GUI out"=w210:refnum<class "Channel.lvclass">)  [unwired: 7 in]
        n85 = call "Write Channel GUI Array.vi"("error in (no error)"=w230, "Channel.lvclass"=w210, "SPARC4_GUI in"=w229) -> ("error out"=w223:errorcluster, "SPARC4_GUI out"=w224:refnum<class "SPARC4_GEI.lvclass">)  [unwired: 7 in]
      }
      event "#Cubes": Value Change {
        n86 = event-data() -> ("NewVal"=w234:u32)  [unwired: 1 in]
        n87 = property on="Cubes done" class="Slide (strict)"("Scale.Maximum"=w234) -> ()  [unwired: 2 in, 2 out]
      }
      event "#Frames": Value Change {
        n88 = event-data() -> ("NewVal"=w239:u16)  [unwired: 1 in]
        n89 = property on="Frames done" class="Slide (strict)"("Scale.Maximum"=w239) -> ()  [unwired: 2 in, 2 out]
      }
      event "Start Iterations": Value Change {
        n90 = event-data() -> ()  [unwired: 1 in, 1 out]
        n91 = call "Read FWCS_ACS_Iterator.lvclass.vi"("error in (no error)"=w263, "SPARC4_GEI in"=w264) -> ("error out"=w258:errorcluster, "FWCS_ACS_Iterator.lvclass"=w259:refnum<class "FWCS_ACS_Iterator.lvclass">, "SPARC4_GEI out"=w255:refnum<class "SPARC4_GEI.lvclass">)  [unwired: 7 in]
        n92 = Build Array("Acquisition configuration", "Acquisition configuration 2", "Acquisition configuration 3", "Acquisition configuration 4", "Acquisition configuration 5", "Acquisition configuration 6") -> (w240:T9)
        n93 = call "Write Array of the iterations config.vi"("error in (no error)"=w258, "Array of the iterations config"=w240, "FWCS_ACS_Iterator in"=w259) -> ("error out"=w256:errorcluster, "FWCS_ACS_Iterator out"=w257:refnum<class "FWCS_ACS_Iterator.lvclass">)  [unwired: 7 in]
        n94 = call "Write Iterations Number.vi"("error in (no error)"=w256, "Iterations Number"="Number of iterations", "FWCS_ACS_Iterator in"=w257) -> ("error out"=w252:errorcluster, "FWCS_ACS_Iterator out"=w253:refnum<class "FWCS_ACS_Iterator.lvclass">)  [unwired: 7 in]
        n95 = call "write state.vi"("error in (no error)"=w252, "State"="SELECT_CONFIGURATION", "FWCS_ACS_Iterator in"=w253) -> ("error out"=w242:errorcluster, "FWCS_ACS_Iterator out"=w245:refnum<class "FWCS_ACS_Iterator.lvclass">)  [unwired: 7 in]
        n96 = call "Write Iterations Done.vi"("error in (no error)"=w242, "Iterations Done"=u16 0, "FWCS_ACS_Iterator in"=w245) -> ("error out"=w243:errorcluster, "FWCS_ACS_Iterator out"=w244:refnum<class "FWCS_ACS_Iterator.lvclass">)  [unwired: 7 in]
        n97 = call "Write FWCS_ACS_Iterator.lvclass.vi"("error in (no error)"=w243, "FWCS_ACS_Iterator.lvclass"=w244, "SPARC4_GEI in"=w255) -> ("error out"=w261:errorcluster, "SPARC4_GEI out"=w262:refnum<class "SPARC4_GEI.lvclass">)  [unwired: 7 in]
      }
      event "stop iterations": Value Change {
        n98 = event-data() -> ()  [unwired: 1 in, 1 out]
        n99 = call "Read FWCS_ACS_Iterator.lvclass.vi"("error in (no error)"=w273, "SPARC4_GEI in"=w274) -> ("error out"=w268:errorcluster, "FWCS_ACS_Iterator.lvclass"=w270:refnum<class "FWCS_ACS_Iterator.lvclass">, "SPARC4_GEI out"=w266:refnum<class "SPARC4_GEI.lvclass">)  [unwired: 7 in]
        n100 = call "Write stop iterations.vi"("error in (no error)"=w268, "stop iterations"="stop iterations", "FWCS_ACS_Iterator in"=w270) -> ("error out"=w267:errorcluster, "FWCS_ACS_Iterator out"=w269:refnum<class "FWCS_ACS_Iterator.lvclass">)  [unwired: 7 in]
        n101 = call "Write FWCS_ACS_Iterator.lvclass.vi"("error in (no error)"=w267, "FWCS_ACS_Iterator.lvclass"=w269, "SPARC4_GEI in"=w266) -> ("error out"=w271:errorcluster, "SPARC4_GEI out"=w272:refnum<class "SPARC4_GEI.lvclass">)  [unwired: 7 in]
      }
      event "Number of iterations": Value Change {
        n102 = event-data() -> ("NewVal"=w275:u16)  [unwired: 1 in]
        n103 = property on="Iterations Done" class="Slide (strict)"("Scale.Maximum"=w275) -> ()  [unwired: 2 in, 2 out]
      }
      event "Sub Image": Value Change {
        w282 = 1024
        n104 = event-data() -> ()  [unwired: 1 in, 1 out]
        n105 = case shown="\"256 x 256\"" "Sub Image" {
          tunnel: [128 256 512 512] -> w286
          frame "256 x 256" {
          }
          frame "512 x 512" {
          }
          frame "1024 x 1024", Default {
          }
          frame "Custom" {
          }
        }
        n106 = case shown="\"Custom\"" "Sub Image" {
          tunnel: [T5."Disabled and Grayed Out" ("Disabled") T5."Enabled" ("Disabled")] -> w289
          frame "1024 x 1024", Default {
          }
          frame "Custom" {
          }
        }
        n107 = Divide(x=w282, y=2) -> (x/y=w285:dbl)
        n108 = Divide(x=w282, y=2) -> (x/y=w284:dbl)
        n109 = Add(x=w285, y=w286) -> (x+y=w278:dbl)
        n110 = Subtract(x=w285, y=w286) -> (x-y=w287:dbl)
        n111 = Subtract(x=w284, y=w286) -> (x-y=w288:dbl)
        n112 = Add(x=w284, y=w286) -> (x+y=w291:dbl)
        n113 = Increment(x=w287) -> (x+1=w290:dbl)
        n114 = Increment(x=w288) -> (x+1=w279:dbl)
        n115 = local write "Initial Cloumn"(w290) -> ()
        n116 = local write "Final Column"(w291) -> ()
        n117 = local write "Initial Line"(w279) -> ()
        n118 = local write "Final Line"(w278) -> ()
        n119 = property on="Initial Line" class="DigNum (strict)"("DisabledEnum"=w289) -> ()  [unwired: 2 in, 2 out]
        n120 = property on="Initial Cloumn" class="DigNum (strict)"("DisabledEnum"=w289) -> ()  [unwired: 2 in, 2 out]
        n121 = property on="Final Line" class="DigNum (strict)"("DisabledEnum"=w289) -> ()  [unwired: 2 in, 2 out]
        n122 = property on="Final Column" class="DigNum (strict)"("DisabledEnum"=w289) -> ()  [unwired: 2 in, 2 out]
        n123 = flat-sequence {
          tunnel: w294 -> [w312]
          tunnel: w295 -> [w313]
          tunnel: [w313] -> w293
          tunnel: [w312] -> w292
          frame #0 {
            w306 = cluster{dbl, dbl} {0.0, 0.0}
            n124 = local read "Initial Cloumn"() -> (w305:u16)
            n125 = local read "Final Column"() -> (w303:u16)
            n126 = local read "Final Line"() -> (w304:u16)
            n127 = local read "Final Line"() -> (w302:u16)
            n128 = Bundle(cluster=w306, w305, w304) -> (w311:cluster{dbl, dbl})
            n129 = Bundle(cluster=w306, w305, w302) -> (w310:cluster{dbl, dbl})
            n130 = Bundle(cluster=w306, w303, w302) -> (w309:cluster{dbl, dbl})
            n131 = Bundle(cluster=w306, w303, w304) -> (w308:cluster{dbl, dbl})
            n132 = Bundle(cluster=w306, w305, w304) -> (w307:cluster{dbl, dbl})
            n133 = Build Array(w311, w310, w309, w308, w307) -> ()  [unwired: 1 out]
          }
        }
      }
      event "Suffix:": Value Change {
        n134 = event-data() -> ()  [unwired: 1 in, 6 out]
        n135 = call "Read Channel GUI Array.vi"("error in (no error)"=w329, "SPARC4_GUI in"=w330) -> ("error out"=w332:errorcluster, "Channel.lvclass"=w333:refnum<class "Channel.lvclass">, "SPARC4_GUI out"=w334:refnum<class "SPARC4_GEI.lvclass">)  [unwired: 7 in]
        n136 = Concatenate Strings("SET SUFFIX ", "Suffix:") -> (w331:string)
        n137 = call "Send Message.vi"("error in (no error)"=w332, "Message"=w331, "Channel GUI in"=w333) -> ("error out"=w315:errorcluster, "Channel GUI out"=w316:refnum<class "Channel.lvclass">)  [unwired: 7 in]
        n138 = call "Read State Machine.lvclass.vi"("error in (no error)"=w315, "Channel GUI in"=w316) -> ("error out"=w322:errorcluster, "State Machine.lvclass"=w317:refnum<class "State Machine.lvclass">, "Channel GUI out"=w323:refnum<class "Channel.lvclass">)  [unwired: 7 in]
        n139 = call-dynamic "Write State.vi"("error in (no error)"=w322, "State"="WAIT_DONE" ("Message"), "State Machine in"=w317) -> ("error out"=w321:errorcluster, "State Machine out"=w318:refnum<class "State Machine.lvclass">)  [unwired: 7 in]
        n140 = call "Write Next State.vi"("error in (no error)"=w321, "Next State"="False" ("Message"), "State Machine in"=w318) -> ("error out"=w320:errorcluster, "State Machine out"=w319:refnum<class "State Machine.lvclass">)  [unwired: 7 in]
        n141 = call "Write State Machine.lvclass.vi"("error in (no error)"=w320, "State Machine.lvclass"=w319, "Channel GUI in"=w323) -> ("error out"=w335:errorcluster, "Channel GUI out"=w314:refnum<class "Channel.lvclass">)  [unwired: 7 in]
        n142 = call "Write Channel GUI Array.vi"("error in (no error)"=w335, "Channel.lvclass"=w314, "SPARC4_GUI in"=w334) -> ("error out"=w327:errorcluster, "SPARC4_GUI out"=w328:refnum<class "SPARC4_GEI.lvclass">)  [unwired: 7 in]
      }
      event "Comment:": Value Change {
        n143 = event-data() -> ()  [unwired: 1 in, 1 out]
        n144 = call "Read Channel GUI Array.vi"("error in (no error)"=w352, "SPARC4_GUI in"=w353) -> ("error out"=w355:errorcluster, "Channel.lvclass"=w356:refnum<class "Channel.lvclass">, "SPARC4_GUI out"=w357:refnum<class "SPARC4_GEI.lvclass">)  [unwired: 7 in]
        n145 = Concatenate Strings("SET COMMENT ", "Comment:") -> (w354:string)
        n146 = call "Send Message.vi"("error in (no error)"=w355, "Message"=w354, "Channel GUI in"=w356) -> ("error out"=w338:errorcluster, "Channel GUI out"=w339:refnum<class "Channel.lvclass">)  [unwired: 7 in]
        n147 = call "Read State Machine.lvclass.vi"("error in (no error)"=w338, "Channel GUI in"=w339) -> ("error out"=w345:errorcluster, "State Machine.lvclass"=w340:refnum<class "State Machine.lvclass">, "Channel GUI out"=w346:refnum<class "Channel.lvclass">)  [unwired: 7 in]
        n148 = call-dynamic "Write State.vi"("error in (no error)"=w345, "State"="WAIT_DONE" ("Message"), "State Machine in"=w340) -> ("error out"=w344:errorcluster, "State Machine out"=w341:refnum<class "State Machine.lvclass">)  [unwired: 7 in]
        n149 = call "Write Next State.vi"("error in (no error)"=w344, "Next State"="False" ("Message"), "State Machine in"=w341) -> ("error out"=w343:errorcluster, "State Machine out"=w342:refnum<class "State Machine.lvclass">)  [unwired: 7 in]
        n150 = call "Write State Machine.lvclass.vi"("error in (no error)"=w343, "State Machine.lvclass"=w342, "Channel GUI in"=w346) -> ("error out"=w358:errorcluster, "Channel GUI out"=w337:refnum<class "Channel.lvclass">)  [unwired: 7 in]
        n151 = call "Write Channel GUI Array.vi"("error in (no error)"=w358, "Channel.lvclass"=w337, "SPARC4_GUI in"=w357) -> ("error out"=w350:errorcluster, "SPARC4_GUI out"=w351:refnum<class "SPARC4_GEI.lvclass">)  [unwired: 7 in]
      }
      event "ZERO": Value Change {
        w378 = FALSE
        n152 = event-data() -> ()  [unwired: 1 in, 3 out]
        n153 = Select(t="zero", s="ZERO", f="") -> (s? t:f=w379:string)
        n154 = call "Read Channel GUI Array.vi"("error in (no error)"=w387, "SPARC4_GUI in"=w388) -> ("error out"=w360:errorcluster, "Channel.lvclass"=w363:refnum<class "Channel.lvclass">, "SPARC4_GUI out"=w380:refnum<class "SPARC4_GEI.lvclass">)  [unwired: 7 in]
        n155 = local write "Suffix:"(w379) -> ()
        n156 = Concatenate Strings("SET OBSTYPE ", w379) -> (w364:string)
        n157 = Concatenate Strings("SET SUFFIX ", w379) -> (w365:string)
        n158 = call "Send Message.vi"("error in (no error)"=w360, "Message"=w364, "Channel GUI in"=w363) -> ("error out"=w361:errorcluster, "Channel GUI out"=w362:refnum<class "Channel.lvclass">)  [unwired: 7 in]
        n159 = call "Send Message.vi"("error in (no error)"=w361, "Message"=w365, "Channel GUI in"=w362) -> ("error out"=w366:errorcluster, "Channel GUI out"=w367:refnum<class "Channel.lvclass">)  [unwired: 7 in]
        n160 = call "Read State Machine.lvclass.vi"("error in (no error)"=w366, "Channel GUI in"=w367) -> ("error out"=w373:errorcluster, "State Machine.lvclass"=w368:refnum<class "State Machine.lvclass">, "Channel GUI out"=w374:refnum<class "Channel.lvclass">)  [unwired: 7 in]
        n161 = call-dynamic "Write State.vi"("error in (no error)"=w373, "State"="WAIT_DONE" ("Message"), "State Machine in"=w368) -> ("error out"=w372:errorcluster, "State Machine out"=w369:refnum<class "State Machine.lvclass">)  [unwired: 7 in]
        n162 = call "Write Next State.vi"("error in (no error)"=w372, "Next State"="False" ("Message"), "State Machine in"=w369) -> ("error out"=w371:errorcluster, "State Machine out"=w370:refnum<class "State Machine.lvclass">)  [unwired: 7 in]
        n163 = call "Write State Machine.lvclass.vi"("error in (no error)"=w371, "State Machine.lvclass"=w370, "Channel GUI in"=w374) -> ("error out"=w389:errorcluster, "Channel GUI out"=w375:refnum<class "Channel.lvclass">)  [unwired: 7 in]
        n164 = call "Write Channel GUI Array.vi"("error in (no error)"=w389, "Channel.lvclass"=w375, "SPARC4_GUI in"=w380) -> ("error out"=w385:errorcluster, "SPARC4_GUI out"=w386:refnum<class "SPARC4_GEI.lvclass">)  [unwired: 7 in]
        n165 = local write "FLAT"(w378) -> ()
        n166 = local write "TEST"(w378) -> ()
        n167 = local write "FOCUS"(w378) -> ()
        n168 = local write "OBJECT"(w378) -> ()
        n169 = local write "DARK"(w378) -> ()
      }
      event "FLAT": Value Change {
        w409 = FALSE
        n170 = event-data() -> ()  [unwired: 1 in, 3 out]
        n171 = Select(t="flat", s="FLAT", f="") -> (s? t:f=w410:string)
        n172 = call "Read Channel GUI Array.vi"("error in (no error)"=w417, "SPARC4_GUI in"=w418) -> ("error out"=w391:errorcluster, "Channel.lvclass"=w392:refnum<class "Channel.lvclass">, "SPARC4_GUI out"=w411:refnum<class "SPARC4_GEI.lvclass">)  [unwired: 7 in]
        n173 = local write "Suffix:"(w410) -> ()
        n174 = Concatenate Strings("SET OBSTYPE ", w410) -> (w396:string)
        n175 = Concatenate Strings("SET SUFFIX ", w410) -> (w395:string)
        n176 = call "Send Message.vi"("error in (no error)"=w391, "Message"=w396, "Channel GUI in"=w392) -> ("error out"=w393:errorcluster, "Channel GUI out"=w394:refnum<class "Channel.lvclass">)  [unwired: 7 in]
        n177 = call "Send Message.vi"("error in (no error)"=w393, "Message"=w395, "Channel GUI in"=w394) -> ("error out"=w397:errorcluster, "Channel GUI out"=w398:refnum<class "Channel.lvclass">)  [unwired: 7 in]
        n178 = call "Read State Machine.lvclass.vi"("error in (no error)"=w397, "Channel GUI in"=w398) -> ("error out"=w404:errorcluster, "State Machine.lvclass"=w399:refnum<class "State Machine.lvclass">, "Channel GUI out"=w405:refnum<class "Channel.lvclass">)  [unwired: 7 in]
        n179 = call-dynamic "Write State.vi"("error in (no error)"=w404, "State"="WAIT_DONE" ("Message"), "State Machine in"=w399) -> ("error out"=w403:errorcluster, "State Machine out"=w400:refnum<class "State Machine.lvclass">)  [unwired: 7 in]
        n180 = call "Write Next State.vi"("error in (no error)"=w403, "Next State"="False" ("Message"), "State Machine in"=w400) -> ("error out"=w402:errorcluster, "State Machine out"=w401:refnum<class "State Machine.lvclass">)  [unwired: 7 in]
        n181 = call "Write State Machine.lvclass.vi"("error in (no error)"=w402, "State Machine.lvclass"=w401, "Channel GUI in"=w405) -> ("error out"=w420:errorcluster, "Channel GUI out"=w419:refnum<class "Channel.lvclass">)  [unwired: 7 in]
        n182 = call "Write Channel GUI Array.vi"("error in (no error)"=w420, "Channel.lvclass"=w419, "SPARC4_GUI in"=w411) -> ("error out"=w415:errorcluster, "SPARC4_GUI out"=w416:refnum<class "SPARC4_GEI.lvclass">)  [unwired: 7 in]
        n183 = local write "ZERO"(w409) -> ()
        n184 = local write "TEST"(w409) -> ()
        n185 = local write "FOCUS"(w409) -> ()
        n186 = local write "OBJECT"(w409) -> ()
        n187 = local write "DARK"(w409) -> ()
      }
      event "DARK": Value Change {
        w441 = FALSE
        n188 = event-data() -> ()  [unwired: 1 in, 3 out]
        n189 = Select(t="dark", s="DARK", f="") -> (s? t:f=w442:string)
        n190 = local write "Suffix:"(w442) -> ()
        n191 = call "Read Channel GUI Array.vi"("error in (no error)"=w449, "SPARC4_GUI in"=w450) -> ("error out"=w422:errorcluster, "Channel.lvclass"=w423:refnum<class "Channel.lvclass">, "SPARC4_GUI out"=w443:refnum<class "SPARC4_GEI.lvclass">)  [unwired: 7 in]
        n192 = Concatenate Strings("SET OBSTYPE ", w442) -> (w427:string)
        n193 = Concatenate Strings("SET SUFFIX ", w442) -> (w426:string)
        n194 = call "Send Message.vi"("error in (no error)"=w422, "Message"=w427, "Channel GUI in"=w423) -> ("error out"=w424:errorcluster, "Channel GUI out"=w425:refnum<class "Channel.lvclass">)  [unwired: 7 in]
        n195 = call "Send Message.vi"("error in (no error)"=w424, "Message"=w426, "Channel GUI in"=w425) -> ("error out"=w429:errorcluster, "Channel GUI out"=w430:refnum<class "Channel.lvclass">)  [unwired: 7 in]
        n196 = call "Read State Machine.lvclass.vi"("error in (no error)"=w429, "Channel GUI in"=w430) -> ("error out"=w436:errorcluster, "State Machine.lvclass"=w431:refnum<class "State Machine.lvclass">, "Channel GUI out"=w437:refnum<class "Channel.lvclass">)  [unwired: 7 in]
        n197 = call-dynamic "Write State.vi"("error in (no error)"=w436, "State"="WAIT_DONE" ("Message"), "State Machine in"=w431) -> ("error out"=w435:errorcluster, "State Machine out"=w432:refnum<class "State Machine.lvclass">)  [unwired: 7 in]
        n198 = call "Write Next State.vi"("error in (no error)"=w435, "Next State"="False" ("Message"), "State Machine in"=w432) -> ("error out"=w434:errorcluster, "State Machine out"=w433:refnum<class "State Machine.lvclass">)  [unwired: 7 in]
        n199 = call "Write State Machine.lvclass.vi"("error in (no error)"=w434, "State Machine.lvclass"=w433, "Channel GUI in"=w437) -> ("error out"=w451:errorcluster, "Channel GUI out"=w428:refnum<class "Channel.lvclass">)  [unwired: 7 in]
        n200 = call "Write Channel GUI Array.vi"("error in (no error)"=w451, "Channel.lvclass"=w428, "SPARC4_GUI in"=w443) -> ("error out"=w447:errorcluster, "SPARC4_GUI out"=w448:refnum<class "SPARC4_GEI.lvclass">)  [unwired: 7 in]
        n201 = local write "ZERO"(w441) -> ()
        n202 = local write "TEST"(w441) -> ()
        n203 = local write "FOCUS"(w441) -> ()
        n204 = local write "OBJECT"(w441) -> ()
        n205 = local write "FLAT"(w441) -> ()
      }
      event "FOCUS": Value Change {
        w472 = FALSE
        n206 = event-data() -> ()  [unwired: 1 in, 3 out]
        n207 = Select(t="focus", s="FOCUS", f="") -> (s? t:f=w473:string)
        n208 = local write "Suffix:"(w473) -> ()
        n209 = call "Read Channel GUI Array.vi"("error in (no error)"=w480, "SPARC4_GUI in"=w481) -> ("error out"=w456:errorcluster, "Channel.lvclass"=w457:refnum<class "Channel.lvclass">, "SPARC4_GUI out"=w474:refnum<class "SPARC4_GEI.lvclass">)  [unwired: 7 in]
        n210 = Concatenate Strings("SET OBSTYPE ", w473) -> (w458:string)
        n211 = Concatenate Strings("SET SUFFIX ", w473) -> (w459:string)
        n212 = call "Send Message.vi"("error in (no error)"=w456, "Message"=w458, "Channel GUI in"=w457) -> ("error out"=w455:errorcluster, "Channel GUI out"=w454:refnum<class "Channel.lvclass">)  [unwired: 7 in]
        n213 = call "Send Message.vi"("error in (no error)"=w455, "Message"=w459, "Channel GUI in"=w454) -> ("error out"=w460:errorcluster, "Channel GUI out"=w461:refnum<class "Channel.lvclass">)  [unwired: 7 in]
        n214 = call "Read State Machine.lvclass.vi"("error in (no error)"=w460, "Channel GUI in"=w461) -> ("error out"=w467:errorcluster, "State Machine.lvclass"=w462:refnum<class "State Machine.lvclass">, "Channel GUI out"=w468:refnum<class "Channel.lvclass">)  [unwired: 7 in]
        n215 = call-dynamic "Write State.vi"("error in (no error)"=w467, "State"="WAIT_DONE" ("Message"), "State Machine in"=w462) -> ("error out"=w466:errorcluster, "State Machine out"=w463:refnum<class "State Machine.lvclass">)  [unwired: 7 in]
        n216 = call "Write Next State.vi"("error in (no error)"=w466, "Next State"="False" ("Message"), "State Machine in"=w463) -> ("error out"=w465:errorcluster, "State Machine out"=w464:refnum<class "State Machine.lvclass">)  [unwired: 7 in]
        n217 = call "Write State Machine.lvclass.vi"("error in (no error)"=w465, "State Machine.lvclass"=w464, "Channel GUI in"=w468) -> ("error out"=w482:errorcluster, "Channel GUI out"=w453:refnum<class "Channel.lvclass">)  [unwired: 7 in]
        n218 = call "Write Channel GUI Array.vi"("error in (no error)"=w482, "Channel.lvclass"=w453, "SPARC4_GUI in"=w474) -> ("error out"=w478:errorcluster, "SPARC4_GUI out"=w479:refnum<class "SPARC4_GEI.lvclass">)  [unwired: 7 in]
        n219 = local write "ZERO"(w472) -> ()
        n220 = local write "TEST"(w472) -> ()
        n221 = local write "OBJECT"(w472) -> ()
        n222 = local write "FLAT"(w472) -> ()
        n223 = local write "FLAT"(w472) -> ()
      }
      event "TEST": Value Change {
        w503 = FALSE
        n224 = event-data() -> ()  [unwired: 1 in, 3 out]
        n225 = Select(t="test", s="TEST", f="") -> (s? t:f=w504:string)
        n226 = call "Read Channel GUI Array.vi"("error in (no error)"=w511, "SPARC4_GUI in"=w512) -> ("error out"=w487:errorcluster, "Channel.lvclass"=w488:refnum<class "Channel.lvclass">, "SPARC4_GUI out"=w505:refnum<class "SPARC4_GEI.lvclass">)  [unwired: 7 in]
        n227 = local write "Suffix:"(w504) -> ()
        n228 = Concatenate Strings("SET OBSTYPE ", w504) -> (w485:string)
        n229 = Concatenate Strings("SET SUFFIX ", w504) -> (w484:string)
        n230 = call "Send Message.vi"("error in (no error)"=w487, "Message"=w485, "Channel GUI in"=w488) -> ("error out"=w490:errorcluster, "Channel GUI out"=w489:refnum<class "Channel.lvclass">)  [unwired: 7 in]
        n231 = call "Send Message.vi"("error in (no error)"=w490, "Message"=w484, "Channel GUI in"=w489) -> ("error out"=w491:errorcluster, "Channel GUI out"=w492:refnum<class "Channel.lvclass">)  [unwired: 7 in]
        n232 = call "Read State Machine.lvclass.vi"("error in (no error)"=w491, "Channel GUI in"=w492) -> ("error out"=w498:errorcluster, "State Machine.lvclass"=w493:refnum<class "State Machine.lvclass">, "Channel GUI out"=w499:refnum<class "Channel.lvclass">)  [unwired: 7 in]
        n233 = call-dynamic "Write State.vi"("error in (no error)"=w498, "State"="WAIT_DONE" ("Message"), "State Machine in"=w493) -> ("error out"=w497:errorcluster, "State Machine out"=w494:refnum<class "State Machine.lvclass">)  [unwired: 7 in]
        n234 = call "Write Next State.vi"("error in (no error)"=w497, "Next State"="False" ("Message"), "State Machine in"=w494) -> ("error out"=w496:errorcluster, "State Machine out"=w495:refnum<class "State Machine.lvclass">)  [unwired: 7 in]
        n235 = call "Write State Machine.lvclass.vi"("error in (no error)"=w496, "State Machine.lvclass"=w495, "Channel GUI in"=w499) -> ("error out"=w513:errorcluster, "Channel GUI out"=w486:refnum<class "Channel.lvclass">)  [unwired: 7 in]
        n236 = call "Write Channel GUI Array.vi"("error in (no error)"=w513, "Channel.lvclass"=w486, "SPARC4_GUI in"=w505) -> ("error out"=w509:errorcluster, "SPARC4_GUI out"=w510:refnum<class "SPARC4_GEI.lvclass">)  [unwired: 7 in]
        n237 = local write "ZERO"(w503) -> ()
        n238 = local write "DARK"(w503) -> ()
        n239 = local write "FOCUS"(w503) -> ()
        n240 = local write "OBJECT"(w503) -> ()
        n241 = local write "FLAT"(w503) -> ()
      }
      event "OBJECT": Value Change {
        w535 = FALSE
        w531 = ""
        n242 = event-data() -> ()  [unwired: 1 in, 3 out]
        n243 = call "Read Channel GUI Array.vi"("error in (no error)"=w540, "SPARC4_GUI in"=w541) -> ("error out"=w515:errorcluster, "Channel.lvclass"=w516:refnum<class "Channel.lvclass">, "SPARC4_GUI out"=w536:refnum<class "SPARC4_GEI.lvclass">)  [unwired: 7 in]
        n244 = local write "Suffix:"(w531) -> ()
        n245 = Concatenate Strings("SET OBSTYPE ", "object") -> (w518:string)
        n246 = Concatenate Strings("SET SUFFIX ", w531) -> (w517:string)
        n247 = call "Send Message.vi"("error in (no error)"=w515, "Message"=w518, "Channel GUI in"=w516) -> ("error out"=w520:errorcluster, "Channel GUI out"=w519:refnum<class "Channel.lvclass">)  [unwired: 7 in]
        n248 = call "Send Message.vi"("error in (no error)"=w520, "Message"=w517, "Channel GUI in"=w519) -> ("error out"=w522:errorcluster, "Channel GUI out"=w523:refnum<class "Channel.lvclass">)  [unwired: 7 in]
        n249 = call "Read State Machine.lvclass.vi"("error in (no error)"=w522, "Channel GUI in"=w523) -> ("error out"=w529:errorcluster, "State Machine.lvclass"=w524:refnum<class "State Machine.lvclass">, "Channel GUI out"=w530:refnum<class "Channel.lvclass">)  [unwired: 7 in]
        n250 = call-dynamic "Write State.vi"("error in (no error)"=w529, "State"="WAIT_DONE" ("Message"), "State Machine in"=w524) -> ("error out"=w528:errorcluster, "State Machine out"=w525:refnum<class "State Machine.lvclass">)  [unwired: 7 in]
        n251 = call "Write Next State.vi"("error in (no error)"=w528, "Next State"="False" ("Message"), "State Machine in"=w525) -> ("error out"=w527:errorcluster, "State Machine out"=w526:refnum<class "State Machine.lvclass">)  [unwired: 7 in]
        n252 = call "Write State Machine.lvclass.vi"("error in (no error)"=w527, "State Machine.lvclass"=w526, "Channel GUI in"=w530) -> ("error out"=w542:errorcluster, "Channel GUI out"=w521:refnum<class "Channel.lvclass">)  [unwired: 7 in]
        n253 = call "Write Channel GUI Array.vi"("error in (no error)"=w542, "Channel.lvclass"=w521, "SPARC4_GUI in"=w536) -> ("error out"=w538:errorcluster, "SPARC4_GUI out"=w539:refnum<class "SPARC4_GEI.lvclass">)  [unwired: 7 in]
        n254 = local write "ZERO"(w535) -> ()
        n255 = local write "TEST"(w535) -> ()
        n256 = local write "FOCUS"(w535) -> ()
        n257 = local write "FLAT"(w535) -> ()
        n258 = local write "DARK"(w535) -> ()
      }
      event "Filter": Value Change {
        n259 = event-data() -> ()  [unwired: 1 in, 3 out]
        n260 = call "Read Filter_Wheel.lvclass.vi"("error in (no error)"=w556, "SPARC4_GEI in"=w555) -> ("error out"=w553:errorcluster, "Filter_Wheel.lvclass"=w554:refnum<class "Filter_Wheel.lvclass">, "SPARC4_GEI out"=w548:refnum<class "SPARC4_GEI.lvclass">)  [unwired: 7 in]
        n261 = call "Write Select Filter.vi"("error in (no error)"=w553, "Select Filter"="Filter", "Filter_Wheel in"=w554) -> ("error out"=w551:errorcluster, "Filter_Wheel out"=w552:refnum<class "Filter_Wheel.lvclass">)  [unwired: 7 in]
        n262 = call "Write State.vi"("error in (no error)"=w551, "State"="SET_FILTER", "Filter_Wheel in"=w552) -> ("error out"=w550:errorcluster, "Filter_Wheel out"=w549:refnum<class "Filter_Wheel.lvclass">)  [unwired: 7 in]
        n263 = call "Write Filter_Wheel.lvclass.vi"("error in (no error)"=w550, "Filter_Wheel.lvclass"=w549, "SPARC4_GEI in"=w548) -> ("error out"=w544:errorcluster, "SPARC4_GEI out"=w545:refnum<class "SPARC4_GEI.lvclass">)  [unwired: 7 in]
      }
      event "Acquisition Mode": Value Change {
        n264 = event-data() -> ("NewVal"=w558:u16)  [unwired: 1 in]
        n265 = case shown="3" w558 {
          tunnel: [T5."Enabled" ("Disabled") T5."Disabled and Grayed Out" ("Disabled")] -> w557
          frame 3 {
          }
          frame 1, Default {
            n266 = local write "#Frames"(u16 1 ("#Frames")) -> ()
          }
        }
        n267 = property on="#Frames" class="DigNum (strict)"("DisabledEnum"=w557) -> ()  [unwired: 2 in, 2 out]
      }
    }
    n268 = Unbundle By Name(w10) -> ("status"=w17:bool)
    n269 = Or(x=w17, y="Stop Application") -> (x .or. y?=w18:bool)
    n270 = call "Erase Message.vi"("error in (no error)"=w10, "SPARC4_GUI in"=w11) -> ("error out"=w13:errorcluster, "SPARC4_GUI out"=w12:refnum<class "SPARC4_GEI.lvclass">)  [unwired: 8 in]
  }
  n271 = Unbundle By Name(w5) -> ("source"=→"Error Message":string)
  n272 = call "End.vi"("SPARC4_GUI in"=w6) -> ("SPARC4_GUI out"=w7:refnum<class "SPARC4_GEI.lvclass">)  [unwired: 9 in, 1 out]
  n273 = flat-sequence {
    tunnel: w7 -> [_]
    frame #0 {
      w569 = u16 1 items=["U"=1, "B"=2, "V"=3, "R"=4, "I"=5, "Clear"=6] ("Current filter")
      w579 = u16 1 items=["U"=1, "B"=2, "V"=3, "R"=4, "I"=5, "Clear"=6] ("Filter")
      w582 = ""
      w581 = FALSE ("Exposing")
      w583 = u16 0 items=["Internal", "External", "N/A", "N/A", "N/A", "N/A", "External Start", "External Exposure (Bulb)", "N/A", "External FVB EM", "Software", "N/A", "External Charge Shifting"] ("Trigger Mode")
      w584 = u16 4 items=["Full Vertical Binning", "Multi-Track", "Random-Track", "Single-Track", "Image"] ("Read Mode")
      w585 = u16 3 items=["Reserved", "Single Scan", "Accumulate", "Kinetic", "Fast Kinetic", "Run till abort", "Reserved", "Reserved", "Reserved", "Time Delayed Integration"] ("Acquisition Mode")
      w590 = u16 0 items=["TTL Low", "TTL High"] ("Shutter TTL")
      w592 = u8 0 items=["  1 MHz", "0.1 MHz"] ("Readout Rate")
      w594 = i16 0 ("Temperature 2")
      w597 = u8 2 items=["Fully Auto", "OPEN", "CLOSED"] ("Shutter Mode")
      w595 = "" ("Command:")
      w599 = u16 1024 ("Final Line")
      w598 = u16 1 ("Initial Cloumn")
      w602 = u8 0 items=["Gain 1", "Gain 2"] ("Pre-amp gain")
      w604 = u16 0 items=["Cooler OFF", "Cooler ON"] ("Cooler ON/OFF")
      w605 = u8 1 items=["Electron Multiplying", "Conventional"] ("EM Mode")
      n274 = local write "Frame exp time (s)"(1.0 ("% Acquired")) -> ()
      n275 = local write "Camera On/Off"(FALSE ("Initialization")) -> ()
      n276 = local write "Exposure Time (s)"(1.0 ("Exposure Time 2")) -> ()
      n277 = local write "Command:"(w595) -> ()
      n278 = local write "Response:"(w595) -> ()
      n279 = local write "Temperature"(20 ("Temperature")) -> ()
      n280 = local write "Exposing"(FALSE ("Exposing")) -> ()
      n281 = local write "#Cubes"(u32 1 ("# Ciclos")) -> ()
      n282 = local write "Shutter Mode"(w597) -> ()
      n283 = local write "Acquisition configuration 6"(T10 {"Select"=FALSE, "Exp Time"=1, "#Frames"=1, "Sufix"="", "Filter"=6} ("Acquisition configuration 6")) -> ()
      n284 = local write "Acquisition configuration 5"(T10 {"Select"=FALSE, "Exp Time"=1, "#Frames"=1, "Sufix"="", "Filter"=5} ("Acquisition configuration 5")) -> ()
      n285 = local write "Acquisition configuration 4"(T10 {"Select"=FALSE, "Exp Time"=1, "#Frames"=1, "Sufix"="", "Filter"=4} ("Acquisition configuration 4")) -> ()
      n286 = local write "Acquisition configuration 3"(T10 {"Select"=FALSE, "Exp Time"=1, "#Frames"=1, "Sufix"="", "Filter"=3} ("Acquisition configuration 3")) -> ()
      n287 = local write "Acquisition configuration 2"(T10 {"Select"=FALSE, "Exp Time"=1, "#Frames"=1, "Sufix"="", "Filter"=2} ("Acquisition configuration 2")) -> ()
      n288 = local write "Acquisition configuration"(T10 {"Select"=FALSE, "Exp Time"=1, "#Frames"=1, "Sufix"="", "Filter"=1} ("Acquisition configuration")) -> ()
      n289 = local write "CCD Status"("" ("CCD Status")) -> ()
      n290 = local write "Last image"(w595) -> ()
      n291 = property on="Cubes done" class="Slide (strict)"("Scale.Maximum"=1.0 ("Scale.Range:Maximum")) -> ()  [unwired: 2 in, 2 out]
      n292 = local write "Cubes done"(u8 1 ("Exposições realizadas")) -> ()
      n293 = property on="Readout Rate" class="Ring (strict)"("Strings []"=string[] ["1 MHz", "0.1 MHz"]) -> ()  [unwired: 2 in, 2 out]
      n294 = local write "Serial Number"(w594) -> ()
      n295 = local write "Temperature"(w594) -> ()
      n296 = local write "Number of iterations"(u16 1 ("Number of iterations")) -> ()
      n297 = local write "Current filter"(w569) -> ()
      n298 = local write "Iterations Done"(u8 0 ("Iterations Done")) -> ()
      n299 = local write "Temperature (ºC)"(i16 20 ("Set temperature")) -> ()
      n300 = local write "EM Gain"(u16 2 ("EM Gain")) -> ()
      n301 = local write "EM Mode"(w605) -> ()
      n302 = local write "Cooler ON/OFF"(w604) -> ()
      n303 = local write "Readout Rate"(w592) -> ()
      n304 = local write "Pre-amp gain"(w602) -> ()
      n305 = local write "Sub Image"(T3."1024 x 1024" ("Sub Image")) -> ()
      n306 = local write "Initial Line"(u16 1 ("Initial Line")) -> ()
      n307 = local write "Final Line"(w599) -> ()
      n308 = local write "Final Column"(w599) -> ()
      n309 = local write "Initial Cloumn"(w598) -> ()
      n310 = local write "Binning"(w598) -> ()
      n311 = local write "#Frames"(u16 1 ("Cube Size  2")) -> ()
      n312 = property on="#Frames" class="DigNum (strict)"("DisabledEnum"=T5."Enabled" ("Disabled")) -> ()  [unwired: 2 in, 2 out]
      n313 = property on="Camera On/Off" class="Bool (strict)"("Colors [4]"=cluster{u32, u32}[] [{1985280, 1985280}]) -> ()  [unwired: 2 in, 2 out]
      n314 = property on="EM Gain" class="DigNum (strict)"("DisabledEnum"=T5."Disabled and Grayed Out" ("Disabled")) -> ()  [unwired: 2 in, 2 out]
      n315 = local write "Suffix:"(w582) -> ()
      n316 = local write "Comment:"(w582) -> ()
      n317 = local write "Frame Tansfer"(TRUE ("Frame Tansfer")) -> ()
      n318 = local write "Shutter TTL"(w590) -> ()
      n319 = local write "Shutter Time"(u16 50 ("Shutter Time")) -> ()
      n320 = local write "Vertical Shift Speed"(u16 3 ("Vertical Shift Speed")) -> ()
      n321 = local write "AD Channel"(u16 0 ("AD Channel")) -> ()
      n322 = local write "Vertical Clock Voltagem"(u16 0 ("Vertical Clock Voltagem")) -> ()
      n323 = local write "Acquisition Mode"(w585) -> ()
      n324 = local write "Read Mode"(w584) -> ()
      n325 = local write "Trigger Mode"(w583) -> ()
      n326 = local write "Filter"(w579) -> ()
      n327 = property on="Temperature" class="DigNum (strict)"("NumText.BGColor"=u32 12369084) -> ()  [unwired: 2 in, 2 out]
      n328 = property on="Frames done" class="Slide (strict)"("Scale.Maximum"=1.0 ("Scale.Range:Maximum")) -> ()  [unwired: 2 in, 2 out]
      n329 = local write "ZERO"(w581) -> ()
      n330 = local write "DARK"(w581) -> ()
      n331 = local write "FLAT"(w581) -> ()
      n332 = local write "FOCUS"(w581) -> ()
      n333 = local write "DARK"(w581) -> ()
      n334 = local write "OBJECT"(w581) -> ()
    }
  }
